vi "Get NbConnections.vi"(8 "error in (no error)":errorcluster, 11 "Server in":refnum<class "Server.lvclass">) -> (0 "error out":errorcluster, 2 "Nb Connections":u32, 3 "Server out":refnum<class "Server.lvclass">)   [LabVIEW 2013, in "MQTT Server.lvlib" / "Server.lvclass"]
uses:
  Server.lvclass
  Server.lvclass/Server.ctl
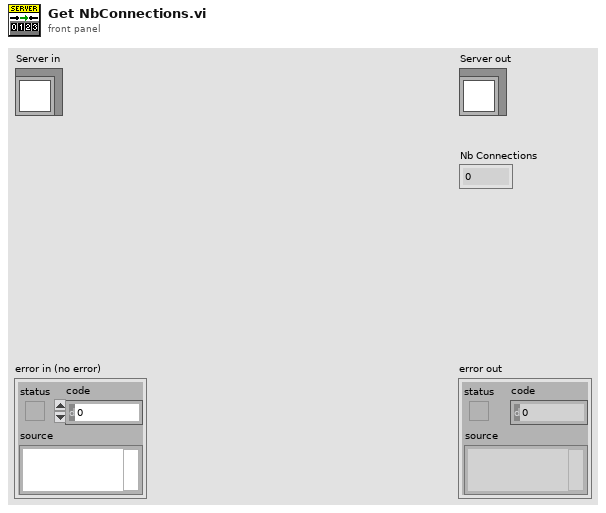
[diagram p1: front panel]
types:
  T1 = typedef "MQTT Server.lvlib/Server.lvclass/SessionRef -- cluster.ctl" = cluster{"ClientID":string, "SessionMailbox":refnum<queue>}
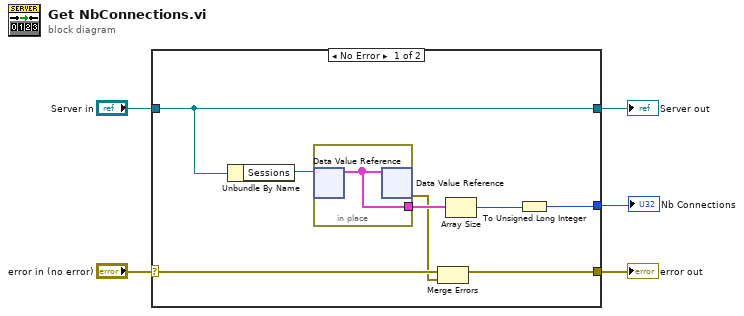
[diagram p0: block diagram]
diagram:
  n1 = case shown="No Error" "error in (no error)" {
    selector: "error in (no error)" -> [w8 w16]
    tunnel: [w6 w16] -> w4
    tunnel: [w13 w15] -> w2
    tunnel: "Server in" -> [w13 w15]
    tunnel: [w9 _] -> w1
    frame No Error {
      n2 = Unbundle By Name(w13) -> ("Sessions"=w12:refnum<data-value>)
      n3 = in-place {
        in-place-border: [w14] -> w10
        n4 = in-place-dvr #1(w12) -> (w14:T1[])  [unwired: 1 out]
        n5 = in-place-dvr #1(w14) -> (w7:errorcluster)  [unwired: 1 out]
      }
      n6 = Merge Errors(w8, w7) -> (w6:errorcluster)
      n7 = Array Size(array=w10) -> (size(s)=w11:i32)
      n8 = To Unsigned Long Integer(number=w11) -> (unsigned 32bit integer=w9:u32)
    }
    frame Error {
    }
  }
  "error out" <- w4
  "Server out" <- w2
  "Nb Connections" <- w1
